vi "GDX_ACC_TiltFilter_Pitch.vi"(8 "Gyro Percent":dbl=75.0, 9 "Gyro Pitch (rad)":dbl, 10 "Accelerometer Pitch (rad)":dbl, 11 "initialize":bool) -> (3 "Filtered Pitch":dbl)   [LabVIEW 2019]
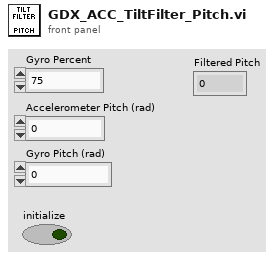
[diagram p1: front panel]
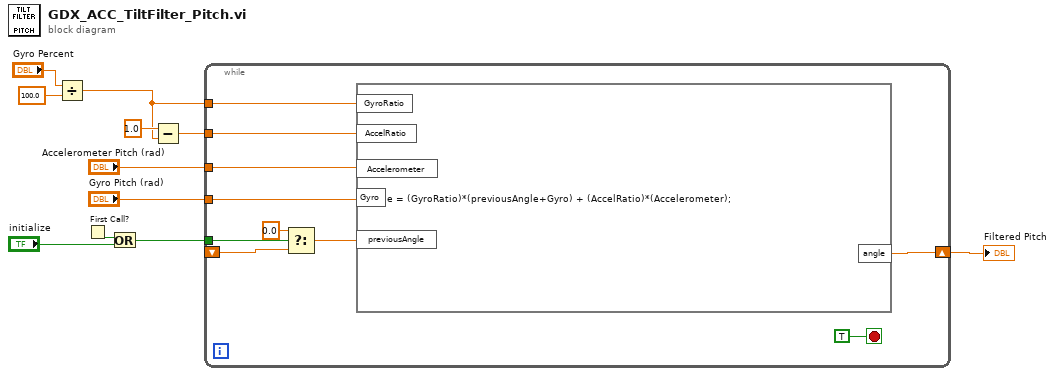
[diagram p0: block diagram]
diagram:
  n1 = Divide(x="Gyro Percent", y=100.0) -> (x/y=w1:dbl)
  n2 = First Call?() -> (First Call?: T/F=w8:bool)
  n3 = Or(x=w8, y="initialize") -> (x .or. y?=w6:bool)
  n4 = Subtract(x=1.0, y=w1) -> (x-y=w4:dbl)
  n5 = while {
    shift-right: [w19] -> w9
    shift-left: _ -> [w15]
    tunnel: "Accelerometer Pitch (rad)" -> [w17]
    tunnel: "Gyro Pitch (rad)" -> [w18]
    tunnel: w1 -> [w20]
    tunnel: w6 -> [w16]
    tunnel: w4 -> [w12]
    stop <- TRUE stop-if-true
    n6 = Select(t=0.0, s=w16, f=w15) -> (s? t:f=w14:dbl)
    n7 = formula code="angle = (GyroRatio)*(previousAngle+Gyro) + (AccelRatio)*(Accelerometer);"("GyroRatio"=w20, "previousAngle"=w14, "Accelerometer"=w17, "Gyro"=w18, "AccelRatio"=w12) -> ("angle"=w19:dbl)
  }
  "Filtered Pitch" <- w9
